vi "Initialize.vi"(8 "error in (no error)":errorcluster, 9 "Reset (True)":bool=TRUE, 10 "ID Query (True)":bool=TRUE, 11 "VISA resource name":refnum<visa-resource-name>) -> (0 "error out":errorcluster, 3 "VISA resource name out":refnum<visa-resource-name>)   [LabVIEW 2012, in "Keysight B2980 Series.lvlib"]
doc: "Establishes communication with the instrument and optionally performs an instrument identification query and/or an instrument reset. It also places the instrument in a default state needed for other instrument driver operations. Therefore, call this VI before calling other instrument driver VIs for this instrument. Generally, you need to call the <b>Initialize</b> VI only once at the beginning of an application."
uses:
  Keysight B2980 Series.lvlib
panel:
  # "(c) 2014 National Instruments.  ALL RIGHTS RESERVED."
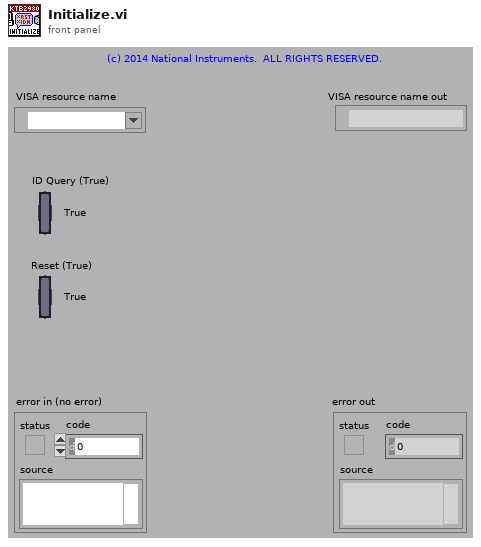
[diagram p1: front panel]
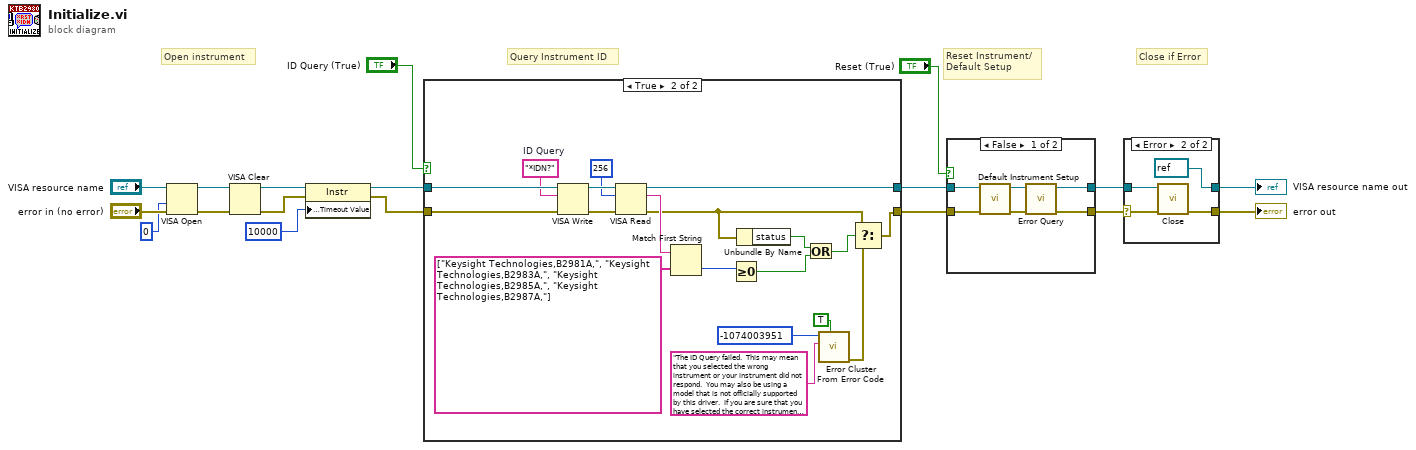
[diagram p0: block diagram]
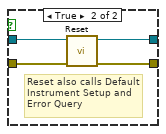
[diagram p3: hidden frame]
diagram:
  # "Close if Error"
  # "Query Instrument ID"
  # "Reset Instrument/\nDefault Setup"
  # "Open instrument"
  n1 = VISA Open(access mode=u32 0, error in (no error)="error in (no error)", VISA resource name="VISA resource name") -> (VISA resource name=w10:refnum<visa-resource-name>, error out=w9:errorcluster)  [unwired: 2 out]
  n2 = VISA Clear(VISA resource name=w10, error in (no error)=w9) -> (VISA resource name out=w8:refnum<visa-resource-name>, error out=w7:errorcluster)
  n3 = property class="Instr"(reference=w8, error in=w7, "General Settings:Timeout Value"=u32 10000) -> (reference out=w2:refnum<visa-resource-name>, error out=w1:errorcluster)
  n4 = case shown="True" "ID Query (True)" {
    tunnel: [w19 w39] -> w17
    tunnel: [w20 w36] -> w18
    tunnel: w2 -> [w20 w37]
    tunnel: w1 -> [w19 w38]
    frame False {
    }
    frame True {
      w31 = "*IDN?"  # ID Query
      n5 = VISA Write(VISA resource name=w37, write buffer=w31, error in (no error)=w38) -> (VISA resource name out=w34:refnum<visa-resource-name>, error out=w33:errorcluster)  [unwired: 1 out]
      n6 = VISA Read(VISA resource name=w34, byte count=u32 256, error in (no error)=w33) -> (VISA resource name out=w36:refnum<visa-resource-name>, read buffer=w35:string, error out=w25:errorcluster)  [unwired: 1 out]
      n7 = Match First String(2:string[] ["Keysight Technologies,B2981A,", "Keysight Technologies,B2983A,", "Keysight Technologies,B2985A,", "Keysight Technologies,B2987A,"] ("string array"), 3:w35) -> (0:w26:i32)  [unwired: 1 out]
      n8 = Greater Or Equal To 0?(x=w26) -> (x >= 0?=w23:bool)
      n9 = Unbundle By Name(w25) -> ("status"=w24:bool)
      n10 = Or(x=w24, y=w23) -> (x .or. y?=w22:bool)
      n11 = call <vilib>:"Error Cluster From Error Code.vi"("show call chain? (False)"=TRUE, "error message (\"\")"="The ID Query failed.  This may mean that you selected the wrong instrument or your instrument did not respond.  You may also be using a model that is not officially supported by this driver.  If you are sure that you have selected the correct instrument and it is responding, try disabling the ID Query." ("Source (VI Name)"), "error code (0)"=-1074003951 ("Code")) -> ("error out"=w30:errorcluster)  [unwired: 1 in, 5 out]
      n12 = Select(t=w25, s=w22, f=w30) -> (s? t:f=w39:errorcluster)
    }
  }
  n13 = case shown="False" "Reset (True)" {
    tunnel: w17 -> [w44 w46]
    tunnel: [w41 w49] -> w3
    tunnel: w18 -> [w45 w47]
    tunnel: [w42 w48] -> w4
    frame False {
      n14 = call "Default Instrument Setup.vi"("error in (no error)"=w44, "VISA resource name"=w45) -> ("error out"=w40:errorcluster, "VISA resource name out"=w43:refnum<visa-resource-name>)  [unwired: 8 out]
      n15 = call "Error Query.vi"("error in (no error)"=w40, "VISA resource name"=w43) -> ("error out"=w41:errorcluster, "VISA resource name out"=w42:refnum<visa-resource-name>)  [unwired: 8 out]
    }
    frame True {
      # "Reset also calls Default Instrument Setup and Error Query"
      n16 = call "Reset.vi"("error in (no error)"=w46, "VISA resource name"=w47) -> ("error out"=w49:errorcluster, "VISA resource name out"=w48:refnum<visa-resource-name>)  [unwired: 8 out]
    }
  }
  n17 = case shown="Error" w3 {
    selector: w3 -> [w50 w53]
    tunnel: w4 -> [w51 w54]
    tunnel: [w51 refnum<visa-resource-name> refnum ("VISA resource name out")] -> w6
    tunnel: [w50 w55] -> w5
    frame No Error {
    }
    frame Error {
      n18 = call "Close.vi"("error in (no error)"=w53, "VISA resource name"=w54) -> ("error out"=w55:errorcluster)  [unwired: 9 out]
    }
  }
  "VISA resource name out" <- w6
  "error out" <- w5
